vi "setOutputMode.vi"(8 "error in (no error)":errorcluster, 9 "pOutputModeStr":string, 11 "pHandle":u32) -> (0 "error out":errorcluster, 3 "return type":i32)   [LabVIEW 2011, in "sbgLabView.lvlib"]
uses:
  sbgLabView.lvlib
  sbgMatLab.dll
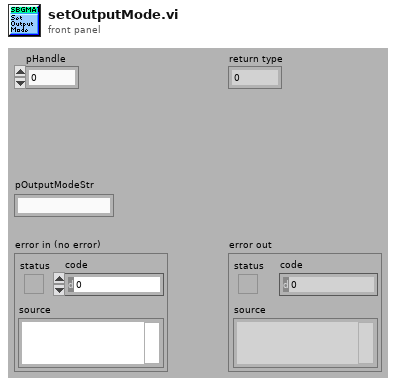
[diagram p1: front panel]
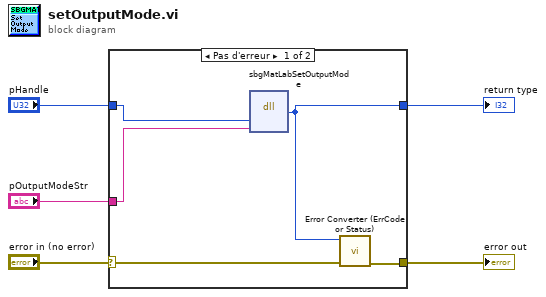
[diagram p0: block diagram]
diagram:
  n1 = case shown="Pas d'erreur" "error in (no error)" {
    selector: "error in (no error)" -> [w8 w11]
    tunnel: [w7 w11] -> w4
    tunnel: [w10 _] -> w3
    tunnel: "pHandle" -> [w9 _]
    tunnel: "pOutputModeStr" -> [w6 _]
    frame No Error {
      n2 = dll-call lib="C:/SBG-Systems/remote/projects/software/projects/labviewExample/sbgLabView/sbgMatLab.*" fn="sbgMatLabSetOutputMode"("pHandle"=w9, "outputModeStr"=w6) -> ("return type"=w10:i32)  [unwired: 5 in, 2 out]
      n3 = call "Error Converter (ErrCode or Status).vi"("error in (no error)"=w8, "error code"=w10) -> ("error out"=w7:errorcluster)  [unwired: 9 in]
    }
    frame Error {
    }
  }
  "return type" <- w3
  "error out" <- w4
